vi "Pre Launch Init.vi"(11 "Nested in":refnum<class "OxxiusLaserController.lvclass">) -> (0 "error out":errorcluster, 3 "Nested out":refnum<class "OxxiusLaserController.lvclass">)   [LabVIEW 2020, in "OxxiusLaserController.lvlib" / "OxxiusLaserController.lvclass"]
doc: "(<B>Filename</B>: Actor Framework.lvlib:Actor.lvclass:Pre Launch Init.vi)\n\nDefines behavior that occurs after the Launch Nested Actor method is invoked but before the actor's Actor Core method begins running.\n\nBy default, this method does nothing. A descendant class may override it to define behavior."
uses:
  OxxiusLaserController.lvclass
  OxxiusLaserController.lvclass/OxxiusLaserController.ctl
  <vilib>/ActorFramework/Actor/Actor.lvclass
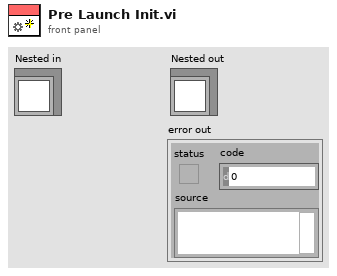
[diagram p1: front panel]
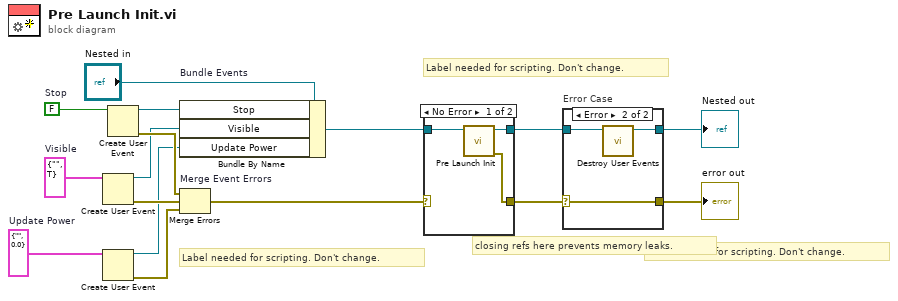
[diagram p0: block diagram]
diagram:
  w3 = cluster{"Label":string, "Value":dbl} {"Label"="", "Value"=0.0}  # Update Power
  w6 = cluster{"Label":string, "Visable?":bool} {"Label"="", "Visable?"=TRUE}  # Visible
  w15 = FALSE  # Stop
  # "Label needed for scripting. Don't change."
  # "Label needed for scripting. Don't change."
  # "Label needed for scripting. Don't change."
  # "closing refs here prevents memory leaks."
  n1 = Create User Event(user event datatype=w6) -> (user event=w5:refnum<user-event>, error out=w4:errorcluster)  [unwired: 1 in]
  n2 = Create User Event(user event datatype=w3) -> (user event=w2:refnum<user-event>, error out=w1:errorcluster)  [unwired: 1 in]
  n3 = Create User Event(user event datatype=w15) -> (user event=w12:refnum<user-event>, error out=w14:errorcluster)  [unwired: 1 in]
  n4 = Bundle By Name "Bundle Events"(cluster="Nested in", "Stop"=w12, "Visible"=w5, "Update Power"=w2) -> (w9:refnum<class "OxxiusLaserController.lvclass">)
  n5 = Merge Errors "Merge Event Errors"(w14, w4, w1) -> (w8:errorcluster)
  n6 = case shown="No Error" w8 {
    selector: w8 -> [_ w21]
    tunnel: [w19 w20] -> w10
    tunnel: w9 -> [w18 w20]
    tunnel: [w17 w21] -> w7
    frame No Error {
      n7 = call-parent "Pre Launch Init.vi"("Actor in"=w18) -> ("error out"=w17:errorcluster, "Actor out"=w19:refnum<class "OxxiusLaserController.lvclass">)  [unwired: 9 in]
    }
    frame Error {
    }
  }
  n8 = case "Error Case" shown="Error" w7 {
    selector: w7 -> [w22 w26]
    tunnel: w10 -> [w23 w25]
    tunnel: [w23 w24] -> w13
    tunnel: [w22 w26] -> w11
    frame No Error {
    }
    frame Error {
      n9 = call "Destroy User Events.vi"("UI Template in"=w25) -> ("UI Template out"=w24:refnum<class "OxxiusLaserController.lvclass">)  [unwired: 10 in]
    }
  }
  "error out" <- w11
  "Nested out" <- w13
